vi "BuildRX.vi"() -> (0 "RX":bool[][](array[boolean]))   [LabVIEW 2018]
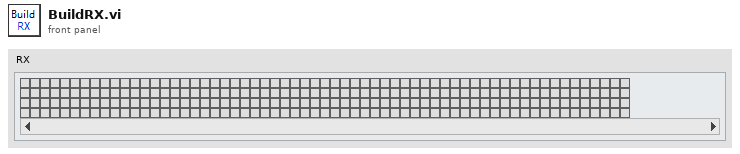
[diagram p1: front panel]
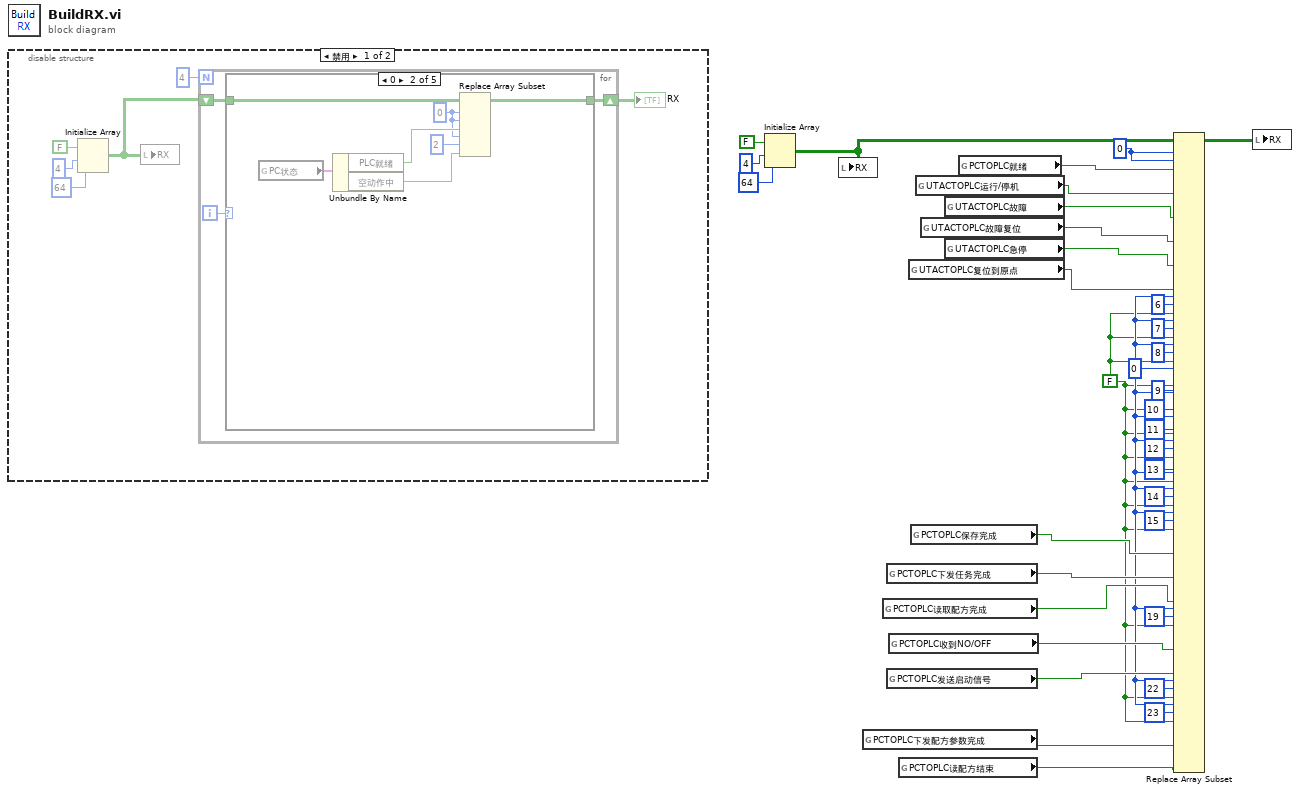
[diagram p0: block diagram]
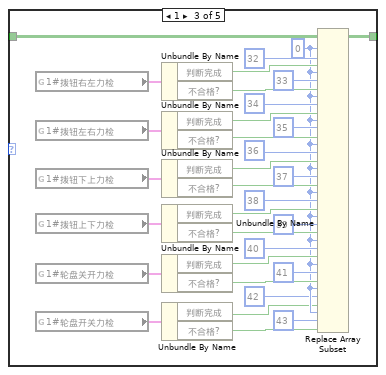
[diagram p3: hidden frame]
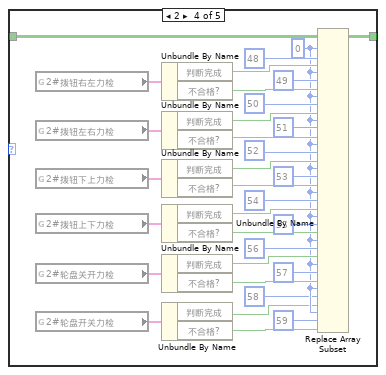
[diagram p4: hidden frame]
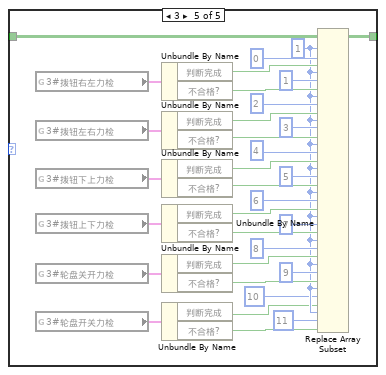
[diagram p5: hidden frame]
diagram:
  w3 = 0 ("索引 (行)")
  w1 = FALSE ("新元素/子数组")
  w33 = 0 ("索引 (行)")
  n1 = disable-structure shown="禁用" {
    frame Disabled {
      n2 = Initialize Array(FALSE, 4 ("维数大小"), 64 ("维数大小")) -> (w40:bool[][])
      n3 = local write "RX"(w40) -> ()
      n4 = for {
        N: 4 -> [_]
        shift-right: [w41] -> w35
        shift-left: w40 -> [w42]
        i -> [w43]
        n5 = case shown="0" w43 {
          tunnel: w42 -> [w44 w50 w83 w116 w149]
          tunnel: [w44 w45 w79 w112 w145] -> w41
          frame -1, Default {
          }
          frame 0 {
            w48 = 0 ("索引 (行)")
            n6 = global read "全局 1.vi" "PC状态"() -> (w51:cluster{"PLC就绪":bool, "空动作中":bool})
            n7 = Unbundle By Name(w51) -> ("PLC就绪"=w49:bool, "空动作中"=w46:bool)
            n8 = Replace Array Subset(array=w50, new element #1=w49, index (row) #1=w48, index (col) #1=w48, new element #2=w46, index (row) #2=w48, index (col) #2=2 ("禁用的索引 (列)")) -> (w45:bool[][])
          }
          frame 1 {
            w57 = 0 ("索引 (行)")
            n9 = global read "全局F结果.vi" "1#拨钮右左力检"() -> (w84:cluster{"判断完成":bool, "不合格?":bool})
            n10 = global read "全局F结果.vi" "1#拨钮左右力检"() -> (w77:cluster{"判断完成":bool, "不合格?":bool})
            n11 = global read "全局F结果.vi" "1#拨钮下上力检"() -> (w72:cluster{"判断完成":bool, "不合格?":bool})
            n12 = global read "全局F结果.vi" "1#拨钮上下力检"() -> (w67:cluster{"判断完成":bool, "不合格?":bool})
            n13 = global read "全局F结果.vi" "1#轮盘关开力检"() -> (w62:cluster{"判断完成":bool, "不合格?":bool})
            n14 = global read "全局F结果.vi" "1#轮盘开关力检"() -> (w54:cluster{"判断完成":bool, "不合格?":bool})
            n15 = Unbundle By Name(w84) -> ("判断完成"=w82:bool, "不合格?"=w80:bool)
            n16 = Unbundle By Name(w77) -> ("判断完成"=w74:bool, "不合格?"=w73:bool)
            n17 = Unbundle By Name(w72) -> ("判断完成"=w69:bool, "不合格?"=w68:bool)
            n18 = Unbundle By Name(w67) -> ("判断完成"=w63:bool, "不合格?"=w64:bool)
            n19 = Unbundle By Name(w62) -> ("判断完成"=w59:bool, "不合格?"=w58:bool)
            n20 = Unbundle By Name(w54) -> ("判断完成"=w52:bool, "不合格?"=w53:bool)
            n21 = Replace Array Subset(array=w83, new element #1=w82, index (row) #1=w57, index (col) #1=32 ("索引 (行)"), new element #2=w80, index (row) #2=w57, index (col) #2=33 ("禁用的索引 (列)"), new element #3=w74, index (row) #3=w57, index (col) #3=34 ("索引 (行)"), new element #4=w73, index (row) #4=w57, index (col) #4=35 ("禁用的索引 (列)"), new element #5=w69, index (row) #5=w57, index (col) #5=36 ("索引 (行)"), new element #6=w68, index (row) #6=w57, index (col) #6=37 ("禁用的索引 (列)"), new element #7=w63, index (row) #7=w57, index (col) #7=38 ("索引 (行)"), new element #8=w64, index (row) #8=w57, index (col) #8=39 ("禁用的索引 (列)"), new element #9=w59, index (row) #9=w57, index (col) #9=40 ("索引 (行)"), new element #10=w58, index (row) #10=w57, index (col) #10=41 ("禁用的索引 (列)"), new element #11=w52, index (row) #11=w57, index (col) #11=42 ("索引 (行)"), new element #12=w53, index (row) #12=w57, index (col) #12=43 ("禁用的索引 (列)")) -> (w79:bool[][])
          }
          frame 2 {
            w90 = 0 ("索引 (行)")
            n22 = global read "全局F结果.vi" "2#拨钮右左力检"() -> (w117:cluster{"判断完成":bool, "不合格?":bool})
            n23 = global read "全局F结果.vi" "2#拨钮左右力检"() -> (w110:cluster{"判断完成":bool, "不合格?":bool})
            n24 = global read "全局F结果.vi" "2#拨钮下上力检"() -> (w105:cluster{"判断完成":bool, "不合格?":bool})
            n25 = global read "全局F结果.vi" "2#拨钮上下力检"() -> (w100:cluster{"判断完成":bool, "不合格?":bool})
            n26 = global read "全局F结果.vi" "2#轮盘关开力检"() -> (w95:cluster{"判断完成":bool, "不合格?":bool})
            n27 = global read "全局F结果.vi" "2#轮盘开关力检"() -> (w87:cluster{"判断完成":bool, "不合格?":bool})
            n28 = Unbundle By Name(w117) -> ("判断完成"=w115:bool, "不合格?"=w113:bool)
            n29 = Unbundle By Name(w110) -> ("判断完成"=w107:bool, "不合格?"=w106:bool)
            n30 = Unbundle By Name(w105) -> ("判断完成"=w102:bool, "不合格?"=w101:bool)
            n31 = Unbundle By Name(w100) -> ("判断完成"=w96:bool, "不合格?"=w97:bool)
            n32 = Unbundle By Name(w95) -> ("判断完成"=w92:bool, "不合格?"=w91:bool)
            n33 = Unbundle By Name(w87) -> ("判断完成"=w85:bool, "不合格?"=w86:bool)
            n34 = Replace Array Subset(array=w116, new element #1=w115, index (row) #1=w90, index (col) #1=48 ("索引 (行)"), new element #2=w113, index (row) #2=w90, index (col) #2=49 ("禁用的索引 (列)"), new element #3=w107, index (row) #3=w90, index (col) #3=50 ("索引 (行)"), new element #4=w106, index (row) #4=w90, index (col) #4=51 ("禁用的索引 (列)"), new element #5=w102, index (row) #5=w90, index (col) #5=52 ("索引 (行)"), new element #6=w101, index (row) #6=w90, index (col) #6=53 ("禁用的索引 (列)"), new element #7=w96, index (row) #7=w90, index (col) #7=54 ("索引 (行)"), new element #8=w97, index (row) #8=w90, index (col) #8=55 ("禁用的索引 (列)"), new element #9=w92, index (row) #9=w90, index (col) #9=56 ("索引 (行)"), new element #10=w91, index (row) #10=w90, index (col) #10=57 ("禁用的索引 (列)"), new element #11=w85, index (row) #11=w90, index (col) #11=58 ("索引 (行)"), new element #12=w86, index (row) #12=w90, index (col) #12=59 ("禁用的索引 (列)")) -> (w112:bool[][])
          }
          frame 3 {
            w123 = 1 ("索引 (行)")
            n35 = global read "全局F结果.vi" "3#拨钮右左力检"() -> (w150:cluster{"判断完成":bool, "不合格?":bool})
            n36 = global read "全局F结果.vi" "3#拨钮左右力检"() -> (w143:cluster{"判断完成":bool, "不合格?":bool})
            n37 = global read "全局F结果.vi" "3#拨钮下上力检"() -> (w138:cluster{"判断完成":bool, "不合格?":bool})
            n38 = global read "全局F结果.vi" "3#拨钮上下力检"() -> (w133:cluster{"判断完成":bool, "不合格?":bool})
            n39 = global read "全局F结果.vi" "3#轮盘关开力检"() -> (w128:cluster{"判断完成":bool, "不合格?":bool})
            n40 = global read "全局F结果.vi" "3#轮盘开关力检"() -> (w120:cluster{"判断完成":bool, "不合格?":bool})
            n41 = Unbundle By Name(w150) -> ("判断完成"=w148:bool, "不合格?"=w146:bool)
            n42 = Unbundle By Name(w143) -> ("判断完成"=w140:bool, "不合格?"=w139:bool)
            n43 = Unbundle By Name(w138) -> ("判断完成"=w135:bool, "不合格?"=w134:bool)
            n44 = Unbundle By Name(w133) -> ("判断完成"=w129:bool, "不合格?"=w130:bool)
            n45 = Unbundle By Name(w128) -> ("判断完成"=w125:bool, "不合格?"=w124:bool)
            n46 = Unbundle By Name(w120) -> ("判断完成"=w118:bool, "不合格?"=w119:bool)
            n47 = Replace Array Subset(array=w149, new element #1=w148, index (row) #1=w123, index (col) #1=0 ("索引 (行)"), new element #2=w146, index (row) #2=w123, index (col) #2=1 ("禁用的索引 (列)"), new element #3=w140, index (row) #3=w123, index (col) #3=2 ("索引 (行)"), new element #4=w139, index (row) #4=w123, index (col) #4=3 ("禁用的索引 (列)"), new element #5=w135, index (row) #5=w123, index (col) #5=4 ("索引 (行)"), new element #6=w134, index (row) #6=w123, index (col) #6=5 ("禁用的索引 (列)"), new element #7=w129, index (row) #7=w123, index (col) #7=6 ("索引 (行)"), new element #8=w130, index (row) #8=w123, index (col) #8=7 ("禁用的索引 (列)"), new element #9=w125, index (row) #9=w123, index (col) #9=8 ("索引 (行)"), new element #10=w124, index (row) #10=w123, index (col) #10=9 ("禁用的索引 (列)"), new element #11=w118, index (row) #11=w123, index (col) #11=10 ("索引 (行)"), new element #12=w119, index (row) #12=w123, index (col) #12=11 ("禁用的索引 (列)")) -> (w145:bool[][])
          }
        }
      }
      "RX" <- w35
    }
    frame Enabled {
    }
  }
  n48 = Initialize Array(FALSE, 4 ("维数大小"), 64 ("维数大小")) -> (w19:bool[][])
  n49 = local write "RX"(w19) -> ()
  n50 = global read "全局 1.vi" "PCTOPLC下发配方参数完成"() -> (w12:bool)
  n51 = global read "全局 1.vi" "PCTOPLC读取配方完成"() -> (w17:bool)
  n52 = global read "全局 1.vi" "PCTOPLC下发任务完成"() -> (w30:bool)
  n53 = global read "全局 1.vi" "PCTOPLC发送启动信号"() -> (w15:bool)
  n54 = global read "全局 1.vi" "PCTOPLC收到NO/OFF"() -> (w18:bool)
  n55 = global read "全局 1.vi" "PCTOPLC读配方结束"() -> (w11:bool)
  n56 = global read "全局 1.vi" "UTACTOPLC复位到原点"() -> (w6:bool)
  n57 = global read "全局 1.vi" "PCTOPLC保存完成"() -> (w31:bool)
  n58 = global read "全局 1.vi" "UTACTOPLC运行/停机"() -> (w10:bool)
  n59 = global read "全局 1.vi" "UTACTOPLC故障复位"() -> (w8:bool)
  n60 = global read "全局 1.vi" "UTACTOPLC故障"() -> (w9:bool)
  n61 = global read "全局 1.vi" "UTACTOPLC急停"() -> (w7:bool)
  n62 = global read "全局 1.vi" "PCTOPLC就绪"() -> (w32:bool)
  n63 = Replace Array Subset(array=w19, new element #1=w32, index (row) #1=w33, index (col) #1=w33, new element #2=w10, new element #3=w9, new element #4=w8, new element #5=w7, new element #6=w6, new element #7=w1, index (row) #7=w3, index (col) #7=6 ("禁用的索引 (列)"), new element #8=w1, index (row) #8=w3, index (col) #8=7 ("禁用的索引 (列)"), new element #9=w1, index (row) #9=w3, index (col) #9=8 ("禁用的索引 (列)"), new element #10=w1, index (row) #10=w3, index (col) #10=9 ("禁用的索引 (列)"), new element #11=w1, index (row) #11=w3, index (col) #11=10 ("禁用的索引 (列)"), new element #12=w1, index (row) #12=w3, index (col) #12=11 ("禁用的索引 (列)"), new element #13=w1, index (row) #13=w3, index (col) #13=12 ("禁用的索引 (列)"), new element #14=w1, index (row) #14=13 ("禁用的索引 (行)"), index (col) #14=w3, new element #15=w1, index (row) #15=w3, index (col) #15=14 ("禁用的索引 (列)"), new element #16=w1, index (row) #16=w3, index (col) #16=15 ("禁用的索引 (列)"), new element #17=w31, new element #18=w30, new element #19=w17, new element #20=w1, index (row) #20=w3, index (col) #20=19 ("禁用的索引 (列)"), new element #21=w18, new element #22=w15, new element #23=w1, index (row) #23=w3, index (col) #23=22 ("禁用的索引 (列)"), new element #24=w1, index (row) #24=w3, index (col) #24=23 ("禁用的索引 (列)"), new element #25=w12, new element #26=w11) -> (w34:bool[][])  [unwired: 24 in]
  n64 = local write "RX"(w34) -> ()
